vi "GetVideoOptionsCodes.vi"(8 "error in (no error)":errorcluster, 11 "CameraSim in":refnum<class "CameraSim.lvclass">) -> (0 "error out":errorcluster, 2 "VideoOptionsCodes":T1 {"ImageTypeCodesList"."Code" format="%.0x"; "VideoResolutionCodesList"."Code" format="%.0x"; "FrameRateCodesList"."Code" format="%.0x"}, 3 "CameraSim out":refnum<class "CameraSim.lvclass">)   [LabVIEW 2020, in "CameraSim.lvlib" / "CameraSim.lvclass"]
uses:
  CameraSim.lvclass
  CameraSim.lvclass/CameraSim.ctl
  ICamera/ICamera/TypeDef/VideoOptionsCodes.ctl
  ICamera/ICamera/ICamera.lvclass
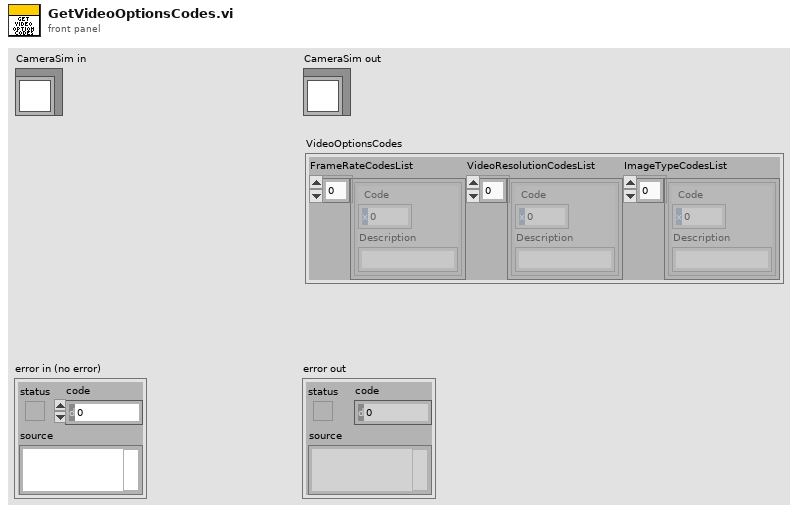
[diagram p1: front panel]
types:
  T1 = typedef "ICamera.lvlib/ICamera.lvclass/VideoOptionsCodes.ctl" = cluster{"FrameRateCodesList":cluster{"Code":u8, "Description":string}[], "VideoResolutionCodesList":cluster{"Code":u8, "Description":string}[], "ImageTypeCodesList":cluster{"Code":u8, "Description":string}[]}
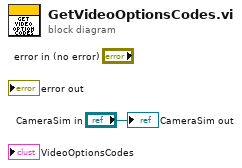
[diagram p0: block diagram]
diagram:
  "CameraSim out" <- "CameraSim in"
